vi "Resample Waveform (single shot).vi"(0 "waveform in":waveform(dbl), 1 "open interval? (F)":bool, 5 "dt":dbl=1.0 format="%.2p", 7 "t0":timestamp=timestamp(-9223372036854775808 s since 1904-01-01) format="%<%.4X>T", 9 "interpolation mode":u16(ring)=1 items=["coerce", "linear", "spline", "FIR filter"], 11 "error in (no error)":errorcluster, 12 "FIR filter specifications":T1={"alias rejection (dB)"=120.0, "normalized bandwidth"=0.4536} {"normalized bandwidth" format="%.4f"; "alias rejection (dB)" format="%.2f"}) -> (4 "resampled waveform out":waveform(dbl), 10 "used t0":timestamp=timestamp(-9223372036854775808 s since 1904-01-01) format="%<%.4X>T", 14 "t0 adjusted warning":bool, 15 "error out":errorcluster)   [LabVIEW 2020, in "NI_MAPro.lvlib"]
doc: "Resamples input waveforms or data according to the user-defined <B>t0</B> and <B>dt</B> values.\n\nWire data to the waveform or data input to determine the polymorphic instance to use or manually select the instance."
uses:
  NI_MAPro.lvlib
  NI_MABase.lvlib
panel:
  # "open"
  # "closed"
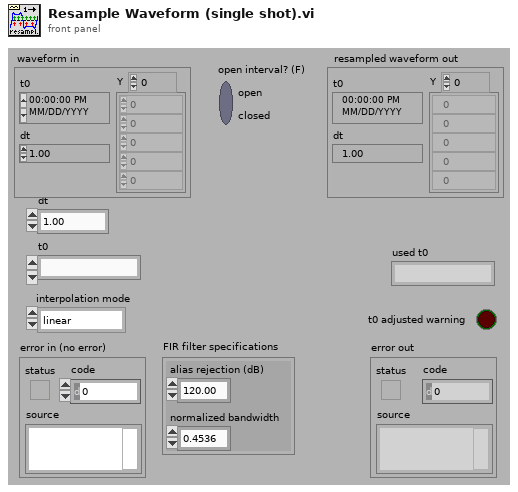
[diagram p1: front panel]
types:
  T1 = cluster{"alias rejection (dB)":dbl, "normalized bandwidth":dbl}
  T2 = cluster{"scaled filter":dbl[], "sub-filter size":i32, "filter max index":i32, "FIR index step":dbl, "half duration":dbl}
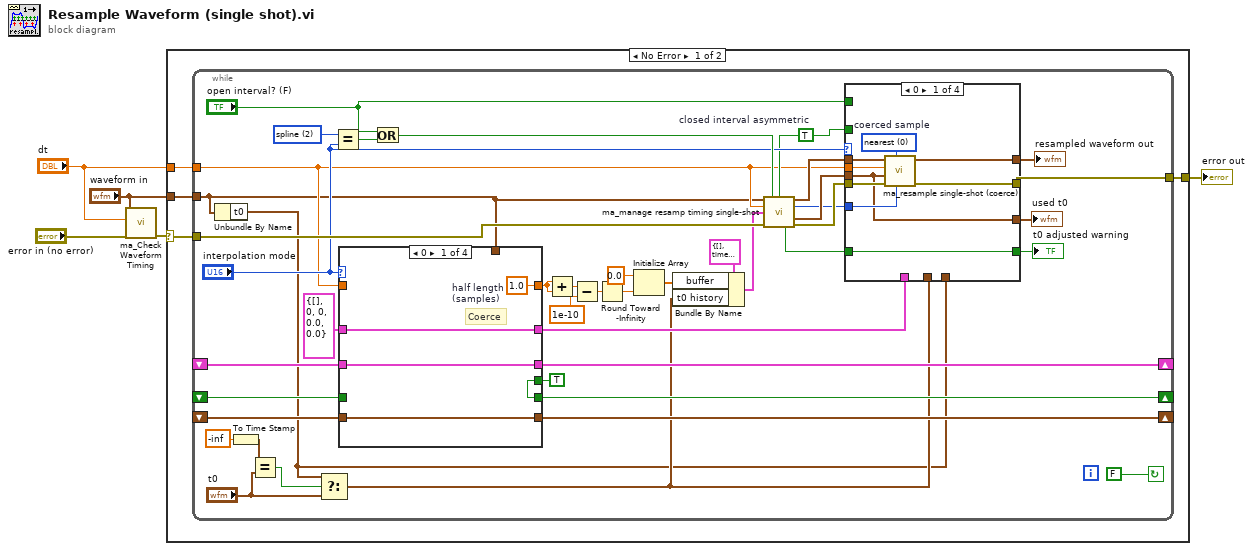
[diagram p0: block diagram]
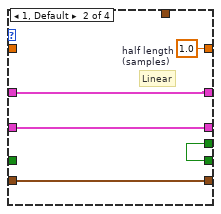
[diagram p2: hidden frame]
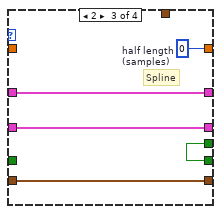
[diagram p3: hidden frame]
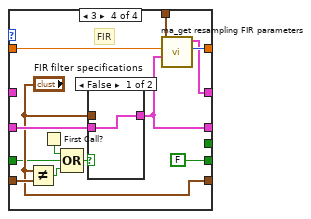
[diagram p4: hidden frame]
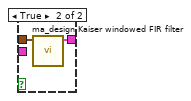
[diagram p5: hidden frame]
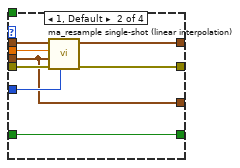
[diagram p6: hidden frame]
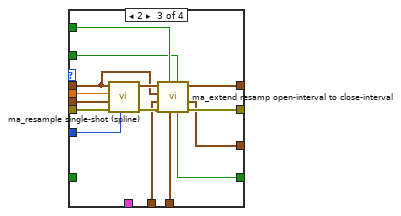
[diagram p7: hidden frame]
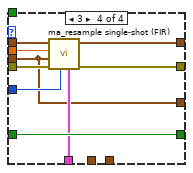
[diagram p8: hidden frame]
diagram:
  n1 = call "ma_Check Waveform Timing.vi"("error in (no error)"="error in (no error)", "dt"="dt", "signal in"="waveform in") -> ("error out"=w3:errorcluster)  [unwired: 7 in, 1 out]
  n2 = case shown="No Error" w3 {
    selector: w3 -> [w8 w125]
    tunnel: [w9 w125] -> w5
    tunnel: "dt" -> [w7 _]
    tunnel: "waveform in" -> [w6 _]
    frame No Error {
      n3 = while {
        tunnel: [w52] -> w9
        tunnel: w8 -> [w51]
        shift-right: [w28] -> _
        shift-left: _ -> [w27]
        shift-right: [w26] -> _
        shift-left: _ -> [w22]
        shift-right: [w24] -> _
        shift-left: _ -> [w23]
        tunnel: w7 -> [w18]
        tunnel: w6 -> [w14]
        stop <- FALSE continue-if-true
        w19 = TRUE  # closed interval asymmetric
        w39 = u16 2 items=["coerce", "linear", "spline", "FIR filter"] ("interpolation mode")
        n4 = Unbundle By Name(w14) -> ("t0"=w13:timestamp)
        n5 = To Time Stamp(1:-inf ("x")) -> (0:w12:timestamp)
        n6 = Equal?(x=w12, y="t0") -> (x = y?=w20:bool)
        n7 = Select(t=w13, s=w20, f="t0") -> (s? t:f=w15:timestamp)
        n8 = Equal?(x=w39, y="interpolation mode") -> (x = y?=w41:bool)
        n9 = case shown="0" "interpolation mode" {
          tunnel: [w57 w62 w67 w80] -> w43
          tunnel: [w56 w61 w66 w79] -> w31
          tunnel: T2 {"scaled filter"=[], "sub-filter size"=0, "filter max index"=0, "FIR index step"=0.0, "half duration"=0.0} ("Filter parameters") -> [w56 w61 w66 _]
          tunnel: w14 -> [_ _ _ w78]
          tunnel: w18 -> [_ _ _ w77]
          tunnel: [w55 w60 w65 w76] -> w28
          tunnel: w27 -> [w55 w60 w65 w75]
          tunnel: [w54 w59 w64 FALSE] -> w26
          tunnel: w22 -> [_ _ _ w70]
          tunnel: TRUE -> [w54 w59 w64 _]
          tunnel: [w53 w58 w63 "FIR filter specifications"] -> w24
          tunnel: w23 -> [w53 w58 w63 w73]
          frame 0 {
            w57 = 1.0  # half length (samples)
            # "Coerce"
          }
          frame 1, Default {
            w62 = 1.0  # half length (samples)
            # "Linear"
          }
          frame 2 {
            w67 = 0  # half length (samples)
            # "Spline"
          }
          frame 3 {
            # "FIR"
            n10 = Not Equal?(x="FIR filter specifications", y=w73) -> (x != y?=w71:bool)
            n11 = First Call?() -> (First Call?: T/F=w68:bool)
            n12 = Compound Arithmetic op=OR(w68, w70, w71) -> (w74:bool)
            n13 = case shown="False" w74 {
              tunnel: [w81 w83] -> w76
              tunnel: "FIR filter specifications" -> [_ w82]
              tunnel: w75 -> [w81 _]
              frame False {
              }
              frame True {
                n14 = call "ma_design Kaiser windowed FIR filter.vi"("FIR filter specifications"=w82) -> ("filter data"=w83:cluster{"h":dbl[], "Max Decimation":dbl})  [unwired: 8 in, 1 out]
              }
            }
            n15 = call "ma_get resampling FIR parameters.vi"("filter info"=w76, "dt"=w77, "Waveform in"=w78) -> ("history size"=w80:i32, "Filter parameters"=w79:T2)  [unwired: 7 in]
          }
        }
        n16 = Or(x="open interval? (F)", y=w41) -> (x .or. y?=w42:bool)
        n17 = Add(x=w43, y=w43) -> (x+y=w46:dbl)
        n18 = Subtract(x=w46, y=1e-10) -> (x-y=w44:dbl)
        n19 = Round Toward -Infinity(1:w44) -> (0:w49:dbl)
        n20 = Initialize Array(0.0 ("element"), w49) -> (w47:dbl[])
        n21 = Bundle By Name(cluster=cluster{"buffer":dbl[], "t0 history":timestamp} {"buffer"=[], "t0 history"=timestamp(0 s since 1904-01-01)} ("state info in"), "buffer"=w47, "t0 history"=w15) -> (w16:cluster{"buffer":dbl[], "t0 history":timestamp})
        n22 = call "ma_manage resamp timing single-shot.vi"("waveform in"=w14, "open interval? (T)"=w42, "closed interval asymmetric"=w19, "dt"=w18, "state info in"=w16, "error in"=w51) -> ("waveform to be processed"=w33:waveform(dbl), "#elements"=w34:i32, "used t0"=w38:timestamp, "t0 adjusted warning"=w36:bool, "error out"=w50:errorcluster)  [unwired: 5 in]
        n23 = case shown="0" "interpolation mode" {
          tunnel: w33 -> [w92 w100 w103 w124]
          tunnel: w34 -> [w85 w94 w104 w118]
          tunnel: w38 -> [w84 w93 w106 w116]
          tunnel: w18 -> [w91 w99 w115 w123]
          tunnel: w50 -> [w90 w98 w114 w122]
          tunnel: [w89 w97 w107 w121] -> w52
          tunnel: [w88 w96 w105 w120] -> w32
          tunnel: [w84 w93 w101 w116] -> w10
          tunnel: w36 -> [w86 w95 _ w119]
          tunnel: [w86 w95 w109 w119] -> w37
          tunnel: "open interval? (F)" -> [_ _ w111 _]
          tunnel: w15 -> [_ _ w110 _]
          tunnel: w13 -> [_ _ w108 _]
          tunnel: w31 -> [_ _ _ w117]
          tunnel: w19 -> [_ _ w102 _]
          frame 0 {
            w87 = u16 0 items=["nearest", "previous", "next"]  # coerced sample
            n24 = call "ma_resample single-shot (coerce).vi"("#elements"=w85, "coerced sample"=w87, "error in"=w90, "t0"=w84, "dt"=w91, "waveform in"=w92) -> ("error out"=w89:errorcluster, "resampled waveform out"=w88:waveform(dbl))  [unwired: 4 in]
          }
          frame 1, Default {
            n25 = call "ma_resample single-shot (linear interpolation).vi"("#elements"=w94, "error in"=w98, "t0"=w93, "dt"=w99, "waveform in"=w100) -> ("error out"=w97:errorcluster, "resampled waveform out"=w96:waveform(dbl))  [unwired: 5 in]
          }
          frame 2 {
            n26 = call "ma_resample single-shot (spline).vi"("#elements"=w104, "error in"=w114, "t0"=w106, "dt"=w115, "waveform in"=w103) -> ("error out"=w113:errorcluster, "resampled waveform out"=w112:waveform(dbl))  [unwired: 3 in, 2 out]
            n27 = call "ma_extend resamp open-interval to close-interval.vi"("closed interval asymmetric"=w102, "t0 WDT in"=w108, "open interval? (T)"=w111, "error in"=w113, "t0 user"=w110, "original waveform in"=w103, "resampled waveform in"=w112) -> ("error out"=w107:errorcluster, "t0 modified"=w101:timestamp, "Waveform out"=w105:waveform(dbl), "t0 adjusted"=w109:bool)  [unwired: 1 in]
          }
          frame 3 {
            n28 = call "ma_resample single-shot (FIR).vi"("Filter parameters"=w117, "#elements"=w118, "error in"=w122, "t0"=w116, "dt"=w123, "waveform in"=w124) -> ("error out"=w121:errorcluster, "resampled waveform out"=w120:waveform(dbl))  [unwired: 4 in]
          }
        }
        "t0 adjusted warning" <- w37
        "used t0" <- w10
        "resampled waveform out" <- w32
      }
    }
    frame Error {
    }
  }
  "error out" <- w5
